vi "Initialize_Array_1D.vi"(9 "Value":i8, 10 "Dimension 1D Array":i32) -> (2 "Initialized Array 1D":i8[](array[numeric]))   [LabVIEW 2018]
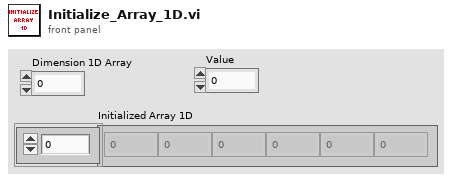
[diagram p1: front panel]
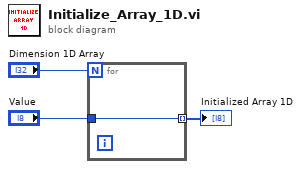
[diagram p0: block diagram]
diagram:
  n1 = for {
    N: "Dimension 1D Array" -> [_]
    tunnel: "Value" -> [w4]
    tunnel: [w4] -> w2 mode=indexing
  }
  "Initialized Array 1D" <- w2
